vi "simple sine gen.vi"(7 "Source":T1={"source"=TRUE, "source type"=FALSE, "Amplitude"=1.0, "Period (steps)"=100.0} {"Amplitude" scale=0.0..1.0; "Period (steps)" scale=1.0..1000.0}) -> (8 "output":dbl)   [LabVIEW 2017]
doc: "This subvi is a one-shot kernal of sine wave generation using an unitialized shift register."
uses:
  typedefs/periodic signal control.ctl
panel:
  out "call counter":dbl
  # "Single Shot Sine Generator Kernel"
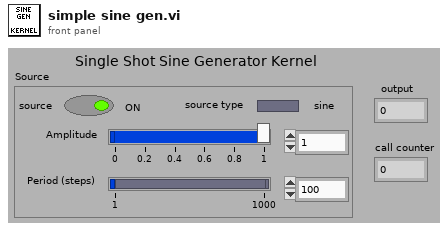
[diagram p1: front panel]
types:
  T1 = typedef "periodic signal control.ctl" = cluster{"source":bool, "source type":bool, "Amplitude":dbl, "Period (steps)":dbl}
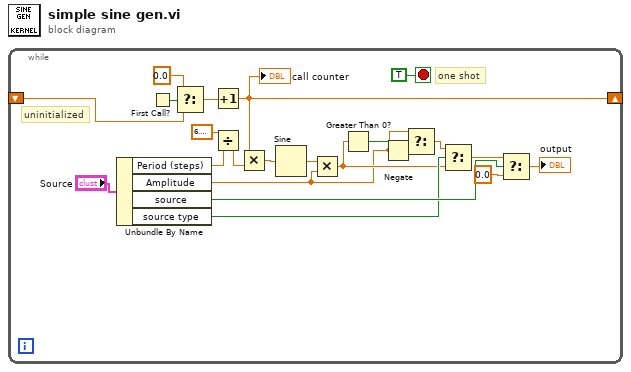
[diagram p0: block diagram]
diagram:
  n1 = while {
    shift-right: [w14] -> _
    shift-left: _ -> [w19]
    stop <- TRUE stop-if-true
    # "uninitialized"
    # "one shot"
    n2 = Unbundle By Name("Source") -> ("Period (steps)"=w12:dbl, "Amplitude"=w2:dbl, "source"=w10:bool, "source type"=w7:bool)
    n3 = First Call?() -> (First Call?: T/F=w20:bool)
    n4 = Select(t=0.0, s=w20, f=w19) -> (s? t:f=w21:dbl)
    n5 = Increment(x=w21) -> (x+1=w14:dbl)
    "call counter" <- w14
    n6 = Divide(x=6.283185307179586, y=w12) -> (x/y=w15:dbl)
    n7 = Multiply(x=w14, y=w15) -> (x*y=w16:dbl)
    n8 = Sine(x=w16) -> (sin(x)=w8:dbl)
    n9 = Multiply(x=w8, y=w2) -> (x*y=w3:dbl)
    n10 = Greater Than 0?(x=w3) -> (x > 0?=w6:bool)
    n11 = Negate(x=w2) -> (-x=w1:dbl)
    n12 = Select(t=w2, s=w6, f=w1) -> (s? t:f=w4:dbl)
    n13 = Select(t=w4, s=w7, f=w3) -> (s? t:f=w5:dbl)
    n14 = Select(t=w5, s=w10, f=0.0) -> (s? t:f=→"output":dbl)
  }
